vi "AutoFillInInfoForPaper1_QuestionTable(SubVI).vi"(11 "Refnum in":T1) -> ()   [LabVIEW 2013]
uses:
  <vilib>/addons/database/Connection.llb/Conn ObjectReference.ctl
  <vilib>/addons/database/NI_Database_API.lvlib
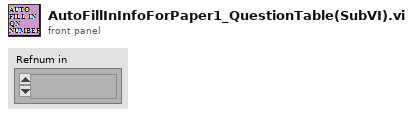
[diagram p1: front panel]
types:
  T1 = typedef "NI_Database_API.lvlib/Conn ObjectReference.ctl" = refnum<k1>
  T2 = cluster{string, string, string, string, string, string, string, string, string, string, string}
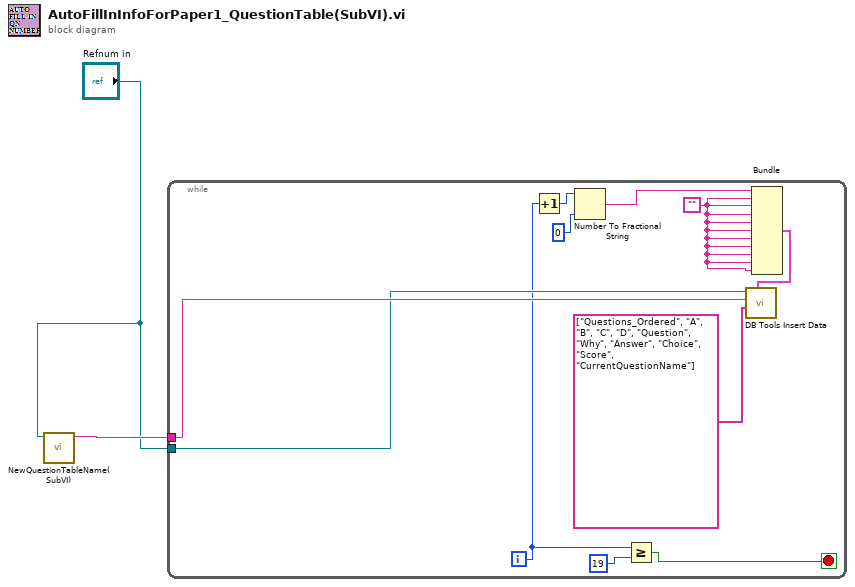
[diagram p0: block diagram]
diagram:
  n1 = call "NewQuestionTableName(SubVI).vi"("connection reference"="Refnum in") -> ("String"=w2:string)  [unwired: 9 in, 1 out]
  n2 = while {
    tunnel: w2 -> [w10]
    tunnel: "Refnum in" -> [w9]
    i -> [w7]
    stop <- w6 stop-if-true
    w3 = ""
    n3 = Increment(x=w7) -> (x+1=w5:i32)
    n4 = Number To Fractional String(number=w5, precision (6)=0) -> (F-format string=w11:string)  [unwired: 2 in]
    n5 = Greater Or Equal?(x=w7, y=19) -> (x >= y?=w6:bool)
    n6 = Bundle(w11, w3, w3, w3, w3, w3, w3, w3, w3, w3, w3) -> (w12:T2)  [unwired: 1 in]
    n7 = call <vilib>:"DB Tools Insert Data.vi"("data"=w12, "columns"=string[] ["Questions_Ordered", "A", "B", "C", "D", "Question", "Why", "Answer", "Choice", "Score", "CurrentQuestionName"], "table"=w10, "connection reference"=w9) -> ()  [unwired: 6 in, 2 out]
  }
